vi "column I64.vi"(8 "error in (no error)":errorcluster, 11 "SQLite3LV Cursor in":refnum<class "cursor.lvclass">) -> (0 "error out":errorcluster, 2 "I64":i64, 3 "SQLite3LV Cursor out":refnum<class "cursor.lvclass">)   [LabVIEW 2014, in "SQLite3LV.lvlib" / "cursor.lvclass"]
uses:
  cursor.lvclass
  cursor.lvclass/cursor.ctl
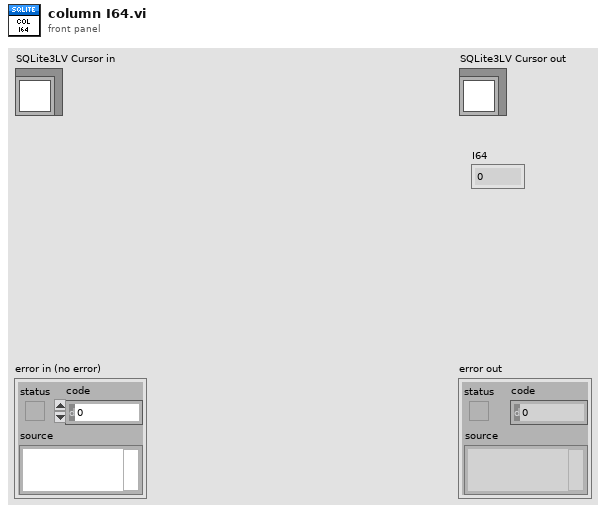
[diagram p1: front panel]
types:
  T1 = typedef "SQLite3LV.lvlib/cursor.lvclass/ctl_active_statement.ctl" = cluster{"ppStmt":i64, "column count":i32, "bind offset":i32, "bind param count":i32, "finished?":bool, "column offset":i32, "column types":i32[]}
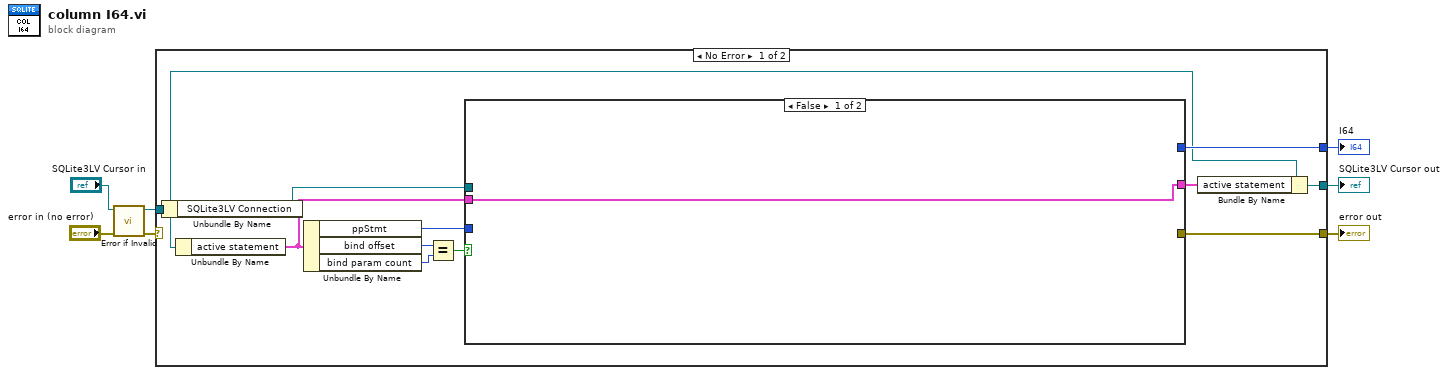
[diagram p0: block diagram]
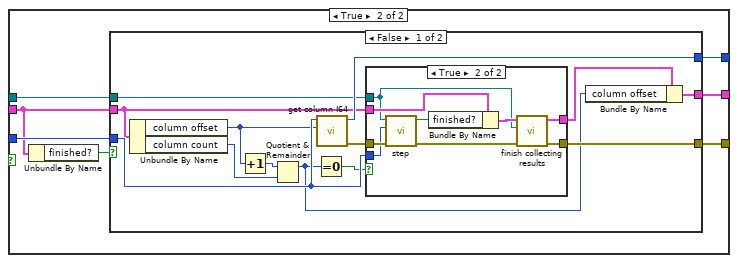
[diagram p2: hidden frame]
diagram:
  n1 = call "Error if Invalid.vi"("error in (no error)"="error in (no error)", "SQLite3LV Cursor in"="SQLite3LV Cursor in") -> ("error out"=w2:errorcluster, "SQLite3LV Cursor out"=w3:refnum<class "cursor.lvclass">)  [unwired: 8 in]
  n2 = case shown="No Error" w2 {
    selector: w2 -> [_ w53]
    tunnel: [w10 w53] -> w6
    tunnel: [w16 w52] -> w7
    tunnel: w3 -> [w17 w52]
    tunnel: [w18 _] -> w5
    frame No Error {
      n3 = Unbundle By Name(w17) -> ("SQLite3LV Connection"=w8:refnum<class "sqlite3.lvclass">)
      n4 = Unbundle By Name(w17) -> ("active statement"=w11:T1)
      n5 = Unbundle By Name(w11) -> ("ppStmt"=w13:i64, "bind offset"=w15:i32, "bind param count"=w14:i32)
      n6 = Equal?(x=w15, y=w14) -> (x = y?=w12:bool)
      n7 = case shown="False" w12 {
        tunnel: w13 -> [_ w26]
        tunnel: w11 -> [w19 w25]
        tunnel: [w19 w23] -> w9
        tunnel: [_ w22] -> w10
        tunnel: [_ w21] -> w18
        tunnel: w8 -> [_ w20]
        frame False {
        }
        frame True {
          n8 = Unbundle By Name(w25) -> ("finished?"=w24:bool)
          n9 = case shown="False" w24 {
            tunnel: w26 -> [w37 _]
            tunnel: w25 -> [w28 w51]
            tunnel: [w38 w51] -> w23
            tunnel: [w36 _] -> w22
            tunnel: [w35 _] -> w21
            tunnel: w20 -> [w29 _]
            frame False {
              n10 = Unbundle By Name(w28) -> ("column offset"=w32:i32, "column count"=w34:i32)
              n11 = Increment(x=w32) -> (x+1=w33:i32)
              n12 = Quotient & Remainder(x=w33, y=w34) -> (x-y*floor(x/y)=w31:i32)  [unwired: 1 out]
              n13 = Equal To 0?(x=w31) -> (x = 0?=w30:bool)
              n14 = call "get column I64.vi"("column index"=w32, "ppStmt"=w37) -> ("error out"=w39:errorcluster, "value"=w35:i64)  [unwired: 8 in]
              n15 = case shown="True" w30 {
                tunnel: w39 -> [w41 w50]
                tunnel: [w41 w49] -> w36
                tunnel: w37 -> [_ w48]
                tunnel: w29 -> [_ w42]
                tunnel: w28 -> [w40 w47]
                tunnel: [w40 w46] -> w27
                frame False {
                }
                frame True {
                  n16 = call "step.vi"("error in (no error)"=w50, "pStmt"=w48, "psqlite"=w42) -> ("error out"=w43:errorcluster, "finished?"=w45:bool)  [unwired: 7 in]
                  n17 = Bundle By Name(cluster=w47, "finished?"=w45) -> (w44:T1)
                  n18 = call "finish collecting results.vi"("error in (no error)"=w43, "psqlite"=w42, "active statement in"=w44) -> ("error out"=w49:errorcluster, "active statement out"=w46:T1)  [unwired: 7 in]
                }
              }
              n19 = Bundle By Name(cluster=w27, "column offset"=w31) -> (w38:T1)
            }
            frame True {
            }
          }
        }
      }
      n20 = Bundle By Name(cluster=w17, "active statement"=w9) -> (w16:refnum<class "cursor.lvclass">)
    }
    frame Error {
    }
  }
  "error out" <- w6
  "SQLite3LV Cursor out" <- w7
  "I64" <- w5
